vi "dfd_Lattice ARMA to TF.vi"(9 "section type":T1(ring), 10 "k":dbl[](array[numeric]) format="%.2f", 11 "v":dbl[](array[numeric]) format="%.2f") -> (2 "denominator":dbl[](array[numeric]) format="%.2f", 3 "numerator":dbl[](array[numeric]) format="%.2f")   [LabVIEW 2017, in "NI_DigFilterLicensed.lvlib"]
uses:
  <vilib>/addons/Digital Filter Design/NI_DigFilterLicensed.lvlib
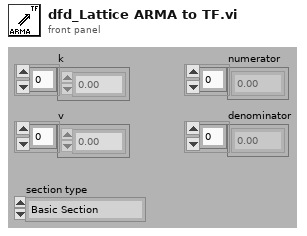
[diagram p1: front panel]
types:
  T1 = enum16{"Basic Section", "One Multiplier Section", "Normalized Section"}
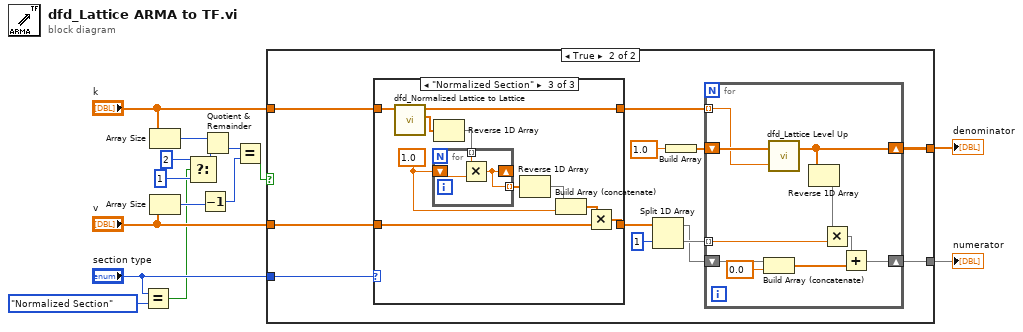
[diagram p0: block diagram]
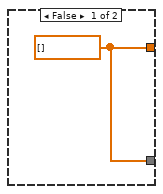
[diagram p2: hidden frame]
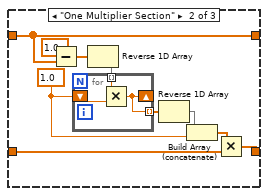
[diagram p4: hidden frame]
diagram:
  n1 = Equal?(x="section type", y=T1."Normalized Section") -> (x = y?=w2:bool)
  n2 = Array Size(array="k") -> (size(s)=w10:i32)
  n3 = Array Size(array="v") -> (size(s)=w11:i32)
  n4 = Select(t=2 ("y"), s=w2, f=1) -> (s? t:f=w1:i32)
  n5 = Decrement(x=w11) -> (x-1=w8:i32)
  n6 = Quotient & Remainder(x=w10, y=w1) -> (floor(x/y)=w9:i32)  [unwired: 1 out]
  n7 = Equal?(x=w9, y=w8) -> (x = y?=w7:bool)
  n8 = case shown="True" w7 {
    tunnel: [w16 w23] -> w15
    tunnel: [w16 w22] -> w14
    tunnel: "k" -> [_ w18]
    tunnel: "v" -> [_ w17]
    tunnel: "section type" -> [_ w19]
    frame False {
      w16 = dbl[] []
    }
    frame True {
      n9 = case shown="\"Normalized Section\"" w19 {
        tunnel: [w29 w31 w45] -> w21
        tunnel: [w30 w38 w52] -> w20
        tunnel: w17 -> [w30 w37 w53]
        tunnel: w18 -> [w29 w31 w46]
        frame "Basic Section", Default {
        }
        frame "One Multiplier Section" {
          w39 = 1.0
          n10 = Subtract(x=1.0, y=w31) -> (x-y=w32:dbl[])
          n11 = Reverse 1D Array(array=w32) -> (reversed array=w36:dbl[])
          n12 = for {
            tunnel: [w41] -> w34 mode=indexing
            tunnel: w36 -> [w43] mode=indexing
            shift-right: [w41] -> _
            shift-left: w39 -> [w42]
            n13 = Multiply(x=w43, y=w42) -> (x*y=w41:dbl)
          }
          n14 = Reverse 1D Array(array=w34) -> (reversed array=w33:dbl[])
          n15 = Build Array (concatenate)(w33, w39) -> (w35:dbl[])
          n16 = Multiply(x=w35, y=w37) -> (x*y=w38:dbl[])
        }
        frame "Normalized Section" {
          w51 = 1.0
          n17 = call <vilib>:"dfd_Normalized Lattice to Lattice.vi"("k & ^k"=w46) -> ("^k [M~1]"=w44:dbl[], "k [M~1]"=w45:dbl[])  [unwired: 9 out]
          n18 = Reverse 1D Array(array=w44) -> (reversed array=w50:dbl[])
          n19 = for {
            tunnel: [w54] -> w48 mode=indexing
            tunnel: w50 -> [w56] mode=indexing
            shift-right: [w54] -> _
            shift-left: w51 -> [w55]
            n20 = Multiply(x=w56, y=w55) -> (x*y=w54:dbl)
          }
          n21 = Reverse 1D Array(array=w48) -> (reversed array=w47:dbl[])
          n22 = Build Array (concatenate)(w47, w51) -> (w49:dbl[])
          n23 = Multiply(x=w49, y=w53) -> (x*y=w52:dbl[])
        }
      }
      n24 = Split 1D Array(array=w20, index=1) -> (first subarray=w24:dbl[], second subarray=w25:dbl[])
      n25 = Build Array(1.0 ("element")) -> (w28:dbl[])
      n26 = for {
        shift-right: [w57] -> w22
        shift-left: w28 -> [w60]
        tunnel: w21 -> [w59] mode=indexing
        tunnel: w25 -> [w66] mode=indexing
        shift-right: [w63] -> w23
        shift-left: w24 -> [w64]
        n27 = Build Array (concatenate)(w64, 0.0) -> (w61:dbl[])
        n28 = call <vilib>:"dfd_Lattice Level Up.vi"("km"=w59, "Bm-1(z)"=w60) -> ("Bm(z)"=w57:dbl[])
        n29 = Reverse 1D Array(array=w57) -> (reversed array=w58:dbl[])
        n30 = Multiply(x=w58, y=w66) -> (x*y=w62:dbl[])
        n31 = Add(x=w62, y=w61) -> (x+y=w63:dbl[])
      }
    }
  }
  "numerator" <- w15
  "denominator" <- w14
